vi "CheckIdleOver23Hrs.vi"() -> ()   [LabVIEW 2012]
uses:
  <vilib>/addons/database/Auxilliary.llb/DB Tools Cursor Type.ctl
  <vilib>/addons/database/Connection.llb/DB Tools Open Connec (Path).vi
  <vilib>/addons/database/Connection.llb/Conn Execute.vi
  <vilib>/addons/database/Recordset.llb/Rec Fetch Recordset Data (R).vi
  <vilib>/addons/database/Recordset.llb/Rec Destroy - Connection.vi
  <vilib>/addons/database/_DB Variant To Data/Database Variant To Data.xnode
  <vilib>/addons/database/NI_Database_API.lvlib
panel:
  out "error out":errorcluster
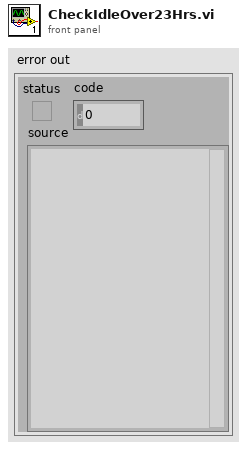
[diagram p1: front panel]
types:
  T1 = typedef "NI_Database_API.lvlib/DB Tools Cursor Type.ctl" = enum16{"forward-only", "keyset", "dynamic", "static"}
  T2 = typedef "NI_Database_API.lvlib/Conn ObjectReference.ctl" = refnum<k1>
  T3 = typedef "NI_Database_API.lvlib/Rec ObjectReference.ctl" = refnum<k1>
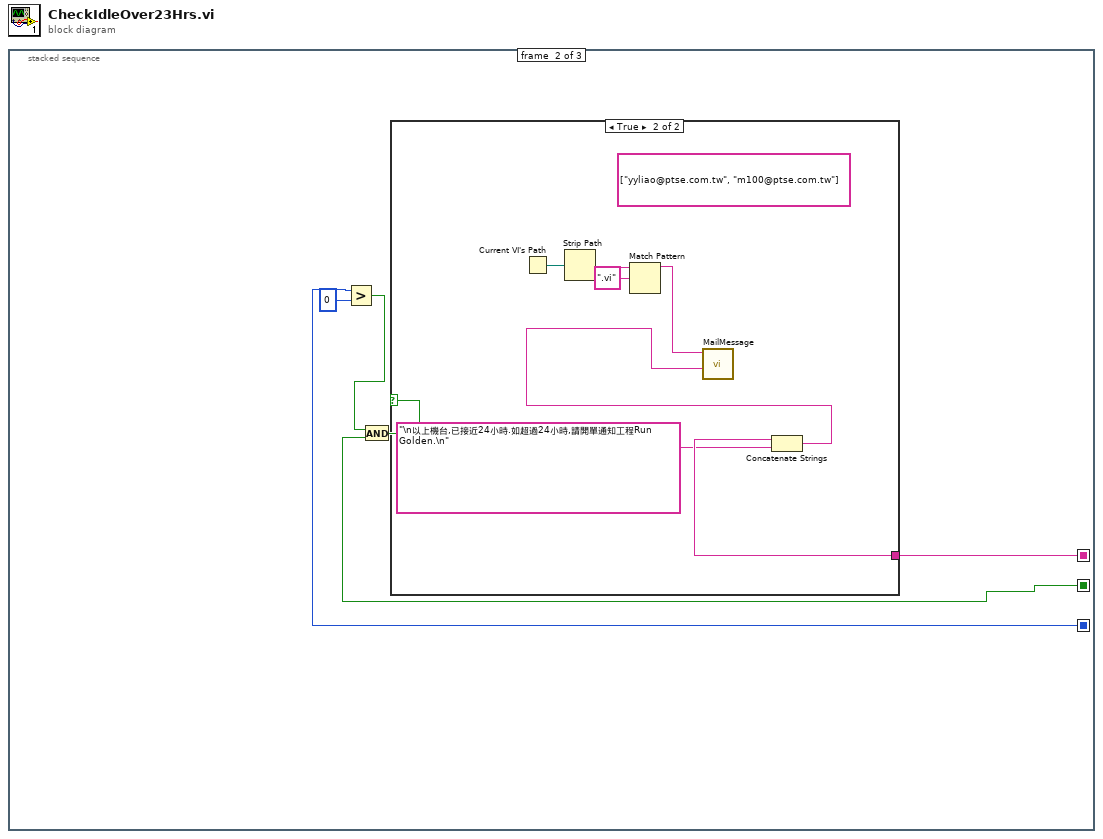
[diagram p0: block diagram]
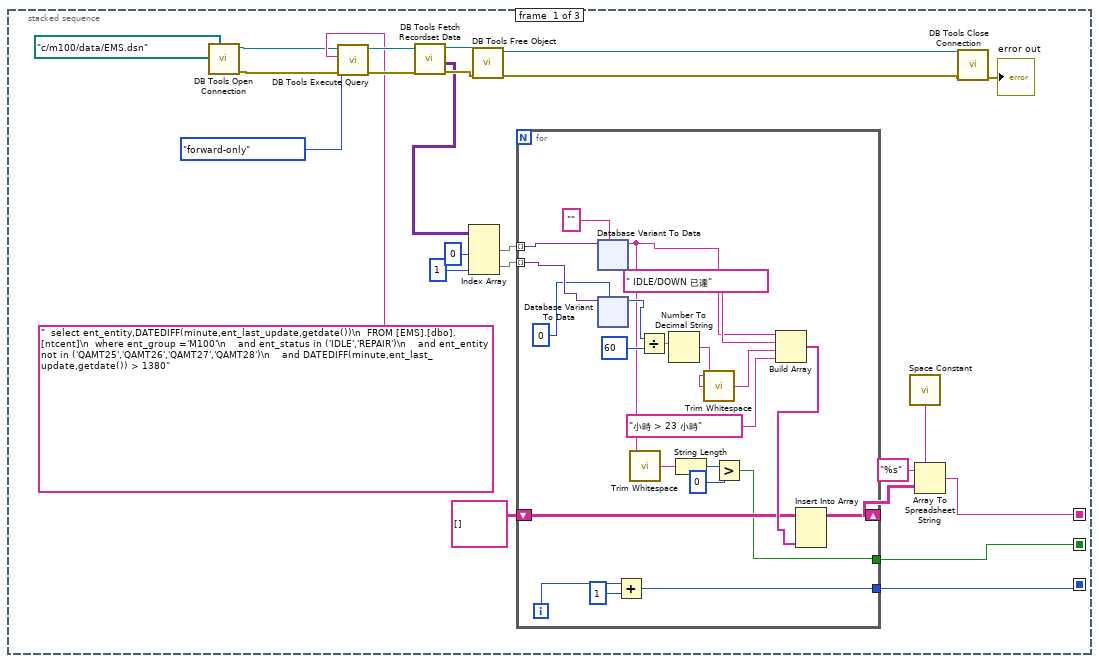
[diagram p2: hidden frame]
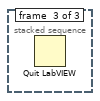
[diagram p4: hidden frame]
diagram:
  n1 = stacked-sequence {
    seq-local: [w10 _ _] -> [_ w116 _]
    seq-local: [w8 _ _] -> [_ w115 _]
    seq-local: [w7 _ _] -> [_ w111 _]
    frame #0 {
      n2 = call-poly <vilib>:"DB Tools Open Connection.vi"("connection information"=path "c:/m100/data/EMS.dsn") -> ("error out"=w5:errorcluster, "connection reference"=w6:T2)  [unwired: 7 in]
      n3 = call-poly <vilib>:"DB Tools Execute Query.vi"("error in (no error)"=w5, "cursor type"=DB_Tools_Cursor_Type."forward-only", "SQL query"="  select ent_entity,DATEDIFF(minute,ent_last_update,getdate())\n  FROM [EMS].[dbo].[ntcent]\n  where ent_group ='M100'\n    and ent_status in ('IDLE','REPAIR')\n    and ent_entity not in ('QAMT25','QAMT26','QAMT27','QAMT28')\n    and DATEDIFF(minute,ent_last_update,getdate()) > 1380", "connection reference"=w6) -> ("error out"=w22:errorcluster, "recordset reference"=w23:T3)  [unwired: 4 in]
      n4 = call-poly <vilib>:"DB Tools Fetch Recordset Data.vi"("error in (no error)"=w22, "recordset reference"=w23) -> ("error out"=w20:errorcluster, "recordset data"=w1:variant[][], "recordset reference out"=w21:T3)  [unwired: 3 in]
      n5 = Index Array(array=w1, index (col) #1=0 ("disabled index (col)"), index (col) #2=1 ("index (col)")) -> (element #1=w14:variant[], element #2=w13:variant[])  [unwired: 2 in]
      n6 = call-poly <vilib>:"DB Tools Free Object.vi"("error in (no error)"=w20, "recordset reference"=w21) -> ("error out"=w2:errorcluster, "connection reference"=w3:T2)  [unwired: 8 in]
      n7 = for {
        tunnel: w14 -> [w46] mode=indexing
        tunnel: w13 -> [w45] mode=indexing
        shift-right: [w42] -> w11
        shift-left: string[][] [] -> [w41]
        tunnel: [w38] -> w8
        tunnel: [w34] -> w7
        i -> [w40]
        n8 = xnode "Database Variant To Data"("database variant"=w46, "type"="") -> ("data"=w27:string)  [unwired: 1 in, 1 out]
        n9 = xnode "Database Variant To Data"("database variant"=w45, "type"=0) -> ("data"=w31:i32)  [unwired: 1 in, 1 out]
        n10 = Add(x=w40, y=1) -> (x+y=w38:i32)
        n11 = call <vilib>:"Trim Whitespace.vi"("string"=w27) -> ("trimmed string"=w37:string)  [unwired: 1 in]
        n12 = Divide(x=w31, y=60) -> (x/y=w29:dbl)
        n13 = Number To Decimal String(number=w29) -> (decimal integer string=w25:string)  [unwired: 1 in]
        n14 = String Length(string=w37) -> (length=w36:i32)
        n15 = call <vilib>:"Trim Whitespace.vi"("string"=w25) -> ("trimmed string"=w26:string)  [unwired: 1 in]
        n16 = Greater?(x=w36, y=0) -> (0:w34:bool)
        n17 = Build Array(w27, " IDLE/DOWN 已達" ("element"), w26, "小時 > 23 小時" ("element")) -> (w43:string[])
        n18 = Insert Into Array(array=w41, new element=w43) -> (w42:string[][])  [unwired: 2 in]
      }
      n19 = call <vilib>:"Space Constant.vi"() -> ("String"=w9:string)
      n20 = Array To Spreadsheet String(delimiter (Tab)=w9, array=w11, 3:"%s" ("format string")) -> (spreadsheet string=w10:string)
      n21 = call <vilib>:"DB Tools Close Connection.vi"("error in (no error)"=w2, "connection reference"=w3) -> ("error out"=→"error out":errorcluster)  [unwired: 5 in]
    }
    frame #1 {
      n22 = Greater?(x=w115, y=0) -> (0:w113:bool)
      n23 = And(x=w113, y=w111) -> (x .and. y?=w112:bool)
      n24 = case shown="True" w112 {
        tunnel: w116 -> [_ w123]
        frame False {
        }
        frame True {
          (unwired) string[] ["yyliao@ptse.com.tw", "m100@ptse.com.tw"] ("recipients")
          n25 = Current VI's Path() -> (path=w121:path)
          n26 = Strip Path(path=w121) -> (name=w120:string)  [unwired: 1 out]
          n27 = Match Pattern(string=w120, regular expression=".vi") -> (before substring=w118:string)  [unwired: 1 in, 3 out]
          n28 = Concatenate Strings(w123, "\n以上機台,已接近24小時.如超過24小時,請開單通知工程Run Golden.\n" ("string")) -> (w117:string)
          n29 = call "MailMessage.vi"("message"=w117, "program"=w118) -> ()  [unwired: 10 in]
        }
      }
    }
    frame #2 {
      n30 = Quit LabVIEW() -> ()  [unwired: 1 in]
    }
  }
